vi "CLD 15 Text String Parsing Solution.vi"(8 "Fehler (Eingang)":T2) -> (0 "Fehler (Ausgang)":T2)   [LabVIEW 2009]
doc: "CLD 15 - Mit diesem VI werden die Datei ausgelesen. Die Daten der Datei werden mit Hilfe von zwei Sub-VIs für die weitere Verwendung analysiert und anschließend formatiert."
uses:
  CLD 15 CSV file data structure.ctl
  <vilib>/Utility/file.llb/Read From Spreadsheet File (string).vi
  <vilib>/Utility/file.llb/Write To Spreadsheet File (string).vi
panel:
  out "Daten":string[][](array[string])
  out "In Datei gespeicherte Daten":string[][](array[string])
  out "Verarbeitete Daten":T1[](array[typedef])
  # "Verarbeitete Daten"
  # "Eingangsdaten"
  # "Ausgangsdaten"
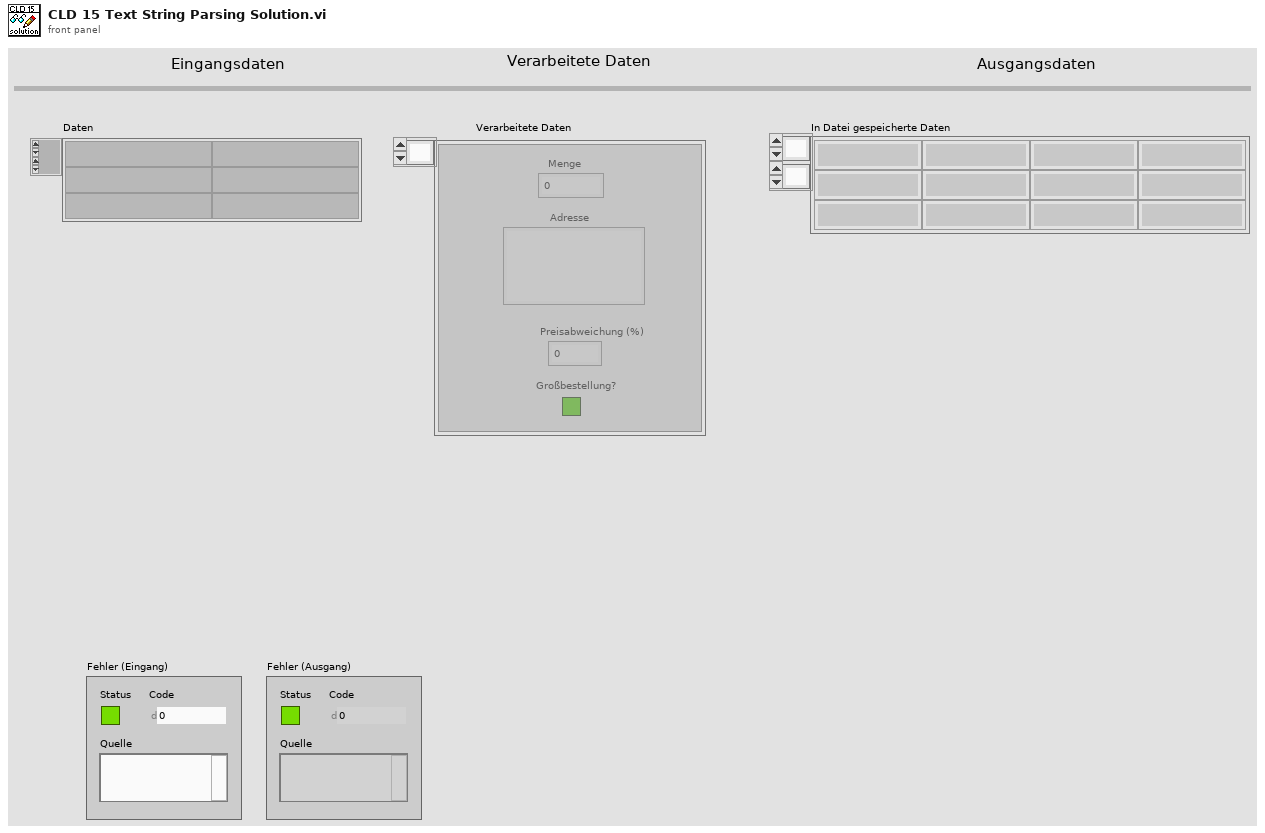
[diagram p1: front panel]
types:
  T1 = typedef "CLD 15 CSV file data structure.ctl" = cluster{"Menge":i32, "Adresse":string, "Preisabweichung (%)":dbl, "Großbestellung?":bool}
  T2 = cluster{"Status":bool, "Code":i32, "Quelle":string}
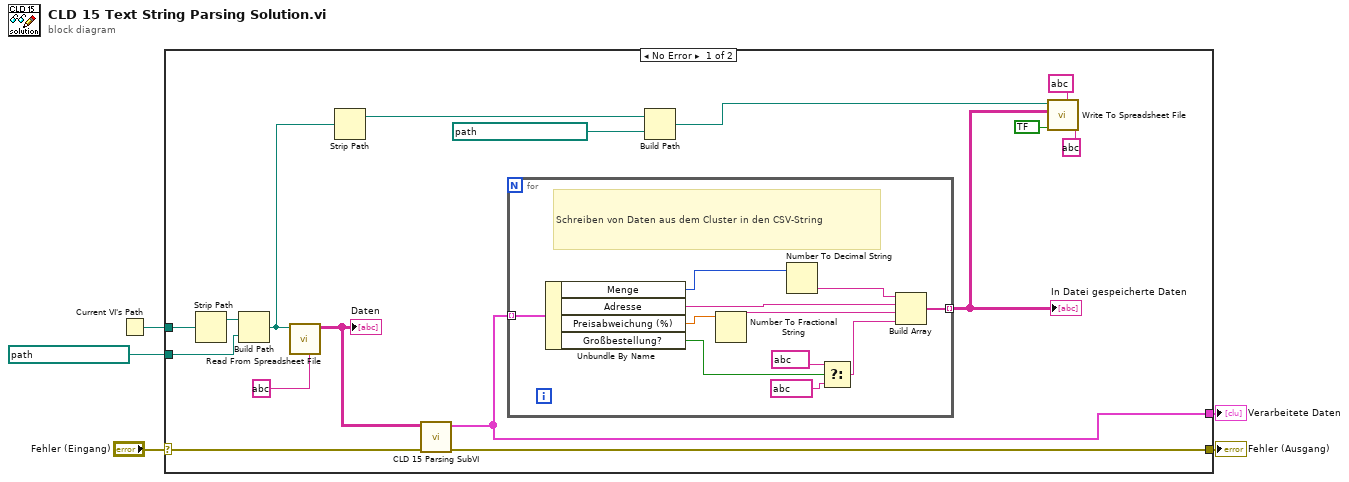
[diagram p0: block diagram]
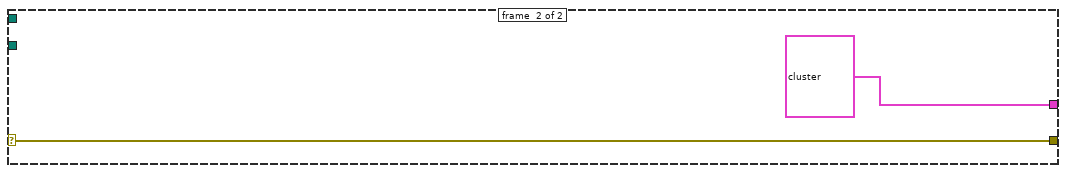
[diagram p2: hidden frame]
diagram:
  n1 = Current VI's Path() -> (path=w4:path)
  n2 = case shown="No Error" "Fehler (Eingang)" {
    selector: "Fehler (Eingang)" -> [w19 w34]
    tunnel: [w7 T1[] ? ("[Daten, Eingang]")] -> w1
    tunnel: path ? -> [w21 _]
    tunnel: w4 -> [w20 _]
    tunnel: [w18 w34] -> w2
    frame #0 {
      n3 = Strip Path(path=w20) -> (stripped path=w17:path)  [unwired: 1 out]
      n4 = Build Path(base path=w17, name or relative path=w21) -> (appended path=w6:path)
      n5 = call-poly <vilib>:"Read From Spreadsheet File.vi"("delimiter (\\t)"=string ? ("Trennzeichen (\\t)"), "file path (dialog if empty)"=w6) -> ("all rows"=w16:string[][])  [unwired: 5 in, 4 out]
      "Daten" <- w16
      n6 = Strip Path(path=w6) -> (stripped path=w11:path)  [unwired: 1 out]
      n7 = call "CLD 15 Parsing SubVI.vi"("Fehler (Eingang)"=w19, "Alle Zeilen (Eingang)"=w16) -> ("Fehler (Ausgang)"=w18:T2, "Daten (Ausgang)"=w7:T1[])  [unwired: 8 in]
      n8 = for {
        tunnel: w7 -> [w32] mode=indexing
        tunnel: [w23] -> w14 mode=indexing
        # "Schreiben von Daten aus dem Cluster in den CSV-String"
        n9 = Unbundle By Name(w32) -> ("Menge"=w31:i32, "Adresse"=w25:string, "Preisabweichung (%)"=w30:dbl, "Großbestellung?"=w29:bool)
        n10 = Number To Fractional String(number=w30) -> (F-format string=w24:string)  [unwired: 3 in]
        n11 = Number To Decimal String(number=w31) -> (decimal integer string=w26:string)  [unwired: 1 in]
        n12 = Select(t=string ?, s=w29, f=string ?) -> (s? t:f=w22:string)
        n13 = Build Array(w26, w25, w24, w22) -> (w23:string[])
      }
      "In Datei gespeicherte Daten" <- w14
      n14 = Build Path(base path=w11, name or relative path=path ?) -> (appended path=w9:path)
      n15 = call-poly <vilib>:"Write To Spreadsheet File.vi"("delimiter (\\t)"=string ? ("Trennzeichen (\\t)"), "format (%s)"=string ? ("Format (%s)"), "append to file? (new file:F)"=bool ? ("An Datei anhängen? (Neue Datei:F)"), "2D data"=w14, "file path (dialog if empty)"=w9) -> ()  [unwired: 3 in, 1 out]
    }
    frame #1 {
    }
  }
  "Fehler (Ausgang)" <- w2
  "Verarbeitete Daten" <- w1
